vi "GetAllDataNoDig.vi"(8 "error in (no error)":errorcluster, 10 "handle in":i32) -> (0 "error out":errorcluster, 2 "handle out":i32, 3 "Data out":T1)   [LabVIEW 2014]
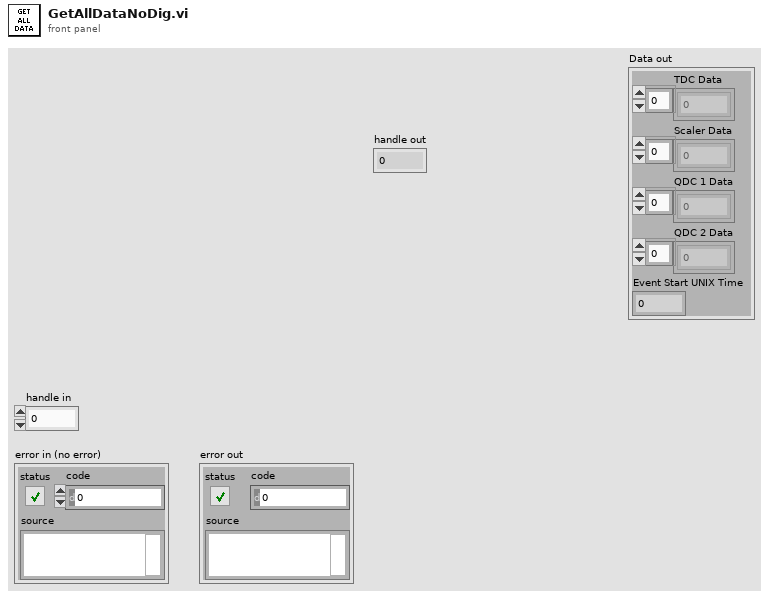
[diagram p1: front panel]
types:
  T1 = cluster{"TDC Data":u32[], "Scaler Data":u32[], "QDC 1 Data":u32[], "QDC 2 Data":u32[], "Event Start UNIX Time":dbl}
  T2 = cluster{"TDC":u32, "Scaler":u32, "QDC 1":u32, "QDC 2":u32, "Digitizer 1":u32, "Digitizer 2":u32}
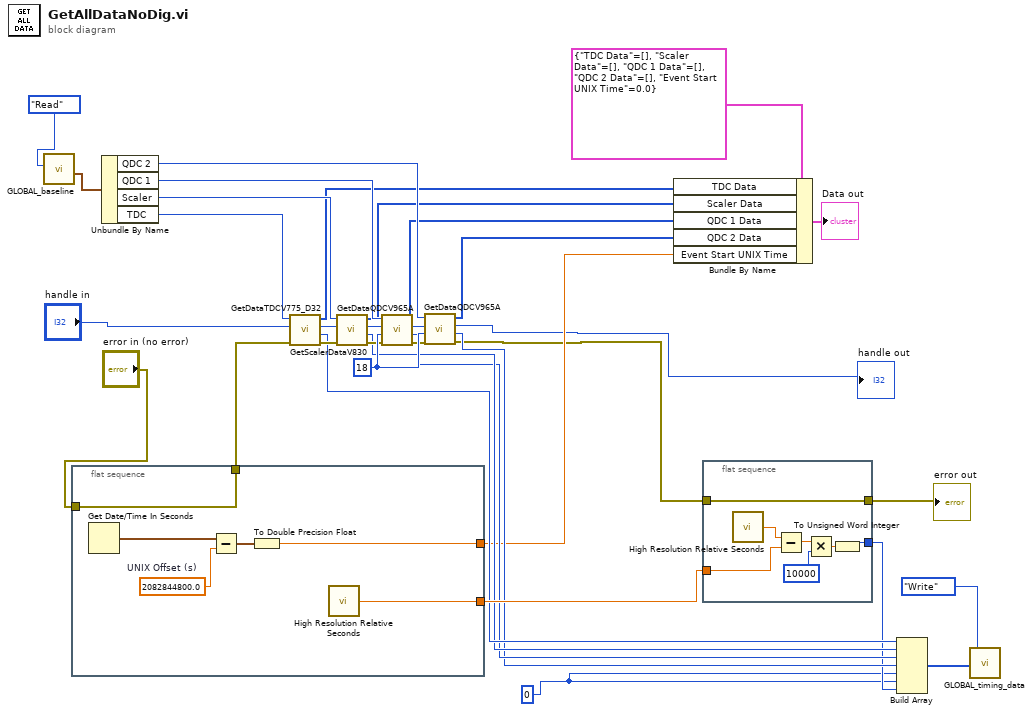
[diagram p0: block diagram]
diagram:
  w2 = u16 0 ("Event Start UNIX Time")
  w35 = 18 ("#samples")
  n1 = call "GLOBAL_baseline.vi"("State"=enum16{"Initialise", "Write", "Read"}."Read") -> ("Addresses Out"=w26:T2)  [unwired: 10 in]
  n2 = flat-sequence {
    tunnel: "error in (no error)" -> [w38]
    tunnel: [w38] -> w15
    tunnel: [w37] -> w5
    tunnel: [w36] -> w13
    frame #0 {
      w41 = 2082844800.0  # UNIX Offset (s)
      n3 = Get Date/Time In Seconds() -> (seconds since 1Jan1904=w39:timestamp)
      n4 = Subtract(x=w39, y=w41) -> (x-y=w40:timestamp)
      n5 = To Double Precision Float(number=w40) -> (double precision float=w37:dbl)
      n6 = call <vilib>:"High Resolution Relative Seconds.vi"() -> ("relative seconds"=w36:dbl)
    }
  }
  n7 = Unbundle By Name(w26) -> ("QDC 2"=w22:u32, "QDC 1"=w23:u32, "Scaler"=w24:u32, "TDC"=w25:u32)
  n8 = call "GetDataTDCV775_D32.vi"("error in (no error)"=w15, "handle in"="handle in", "VME Base Address"=w25) -> ("error out"=w29:errorcluster, "Time Elapsed"=w12:u16, "handle out"=w30:i32, "Array"=w20:u32[])  [unwired: 5 in]
  n9 = call "GetScalerDataV830.vi"("error in (no error)"=w29, "handle in"=w30, "VME Base Address"=w24) -> ("error out"=w31:errorcluster, "Time Elapsed"=w11:u16, "handle out"=w32:i32, "Buff"=w19:u32[])  [unwired: 5 in]
  n10 = call "GetDataQDCV965A.vi"("error in (no error)"=w31, "#samples"=w35, "handle in"=w32, "VME module Base Address"=w23) -> ("error out"=w33:errorcluster, "Time Elapsed"=w10:u16, "handle out"=w34:i32, "Data"=w18:u32[])  [unwired: 4 in]
  n11 = call "GetDataQDCV965A.vi"("error in (no error)"=w33, "#samples"=w35, "handle in"=w34, "VME module Base Address"=w22) -> ("error out"=w3:errorcluster, "Time Elapsed"=w9:u16, "handle out"=→"handle out":i32, "Data"=w17:u32[])  [unwired: 4 in]
  n12 = Bundle By Name(cluster=T1 {"TDC Data"=[], "Scaler Data"=[], "QDC 1 Data"=[], "QDC 2 Data"=[], "Event Start UNIX Time"=0.0}, "TDC Data"=w20, "Scaler Data"=w19, "QDC 1 Data"=w18, "QDC 2 Data"=w17, "Event Start UNIX Time"=w5) -> (→"Data out":T1)
  n13 = flat-sequence {
    tunnel: w3 -> [w48]
    tunnel: [w48] -> w14
    tunnel: w13 -> [w46]
    tunnel: [w42] -> w8
    frame #0 {
      n14 = call <vilib>:"High Resolution Relative Seconds.vi"() -> ("relative seconds"=w47:dbl)
      n15 = Subtract(x=w47, y=w46) -> (x-y=w45:dbl)
      n16 = Multiply(x=w45, y=u16 10000) -> (x*y=w43:dbl)
      n17 = To Unsigned Word Integer(number=w43) -> (unsigned 16bit integer=w42:u16)
    }
  }
  n18 = Build Array(w12, w11, w10, w9, w2, w2, w8) -> (w7:u16[])
  n19 = call "GLOBAL_timing_data.vi"("Data in"=w7, "State"=enum16{"Initialise", "Write", "Read"}."Write") -> ()  [unwired: 2 in, 2 out]
  "error out" <- w14
